vi "test-AsyncMessageWithReplyWithGlobalVariable.vi"(8 "error in (no error)":errorcluster, 11 "TestCase in":refnum<class "testcase-CSMMessage.lvclass">) -> (0 "error out":errorcluster, 3 "TestCase out":refnum<class "testcase-CSMMessage.lvclass">)   [LabVIEW 2017, in "testcase-CSMMessage.lvclass"]
uses:
  testcase-CSMMessage.lvclass
  C:/Program Files (x86)/National Instruments/LabVIEW 2017/vi.lib/addons/_JKI Toolkits/VI Tester/TestCase.llb/TestCase.lvclass
  src/user.lib/_NEVSTOP/Communicable State Machine(CSM)/Communicable State Machine.lvlib
  CSM/Global-TestcaseCSM.vi
  CSM/CSM-Testcase.lvlib
  <vilib>/addons/_JKI Toolkits/VI Tester/TestCase.llb/TestCase.lvclass
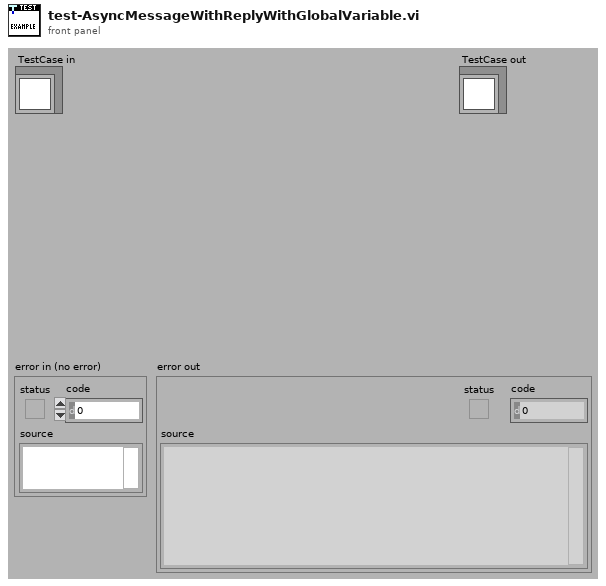
[diagram p1: front panel]
types:
  T1 = cluster{"Arguments":string, "Response":string, "error":errorcluster}
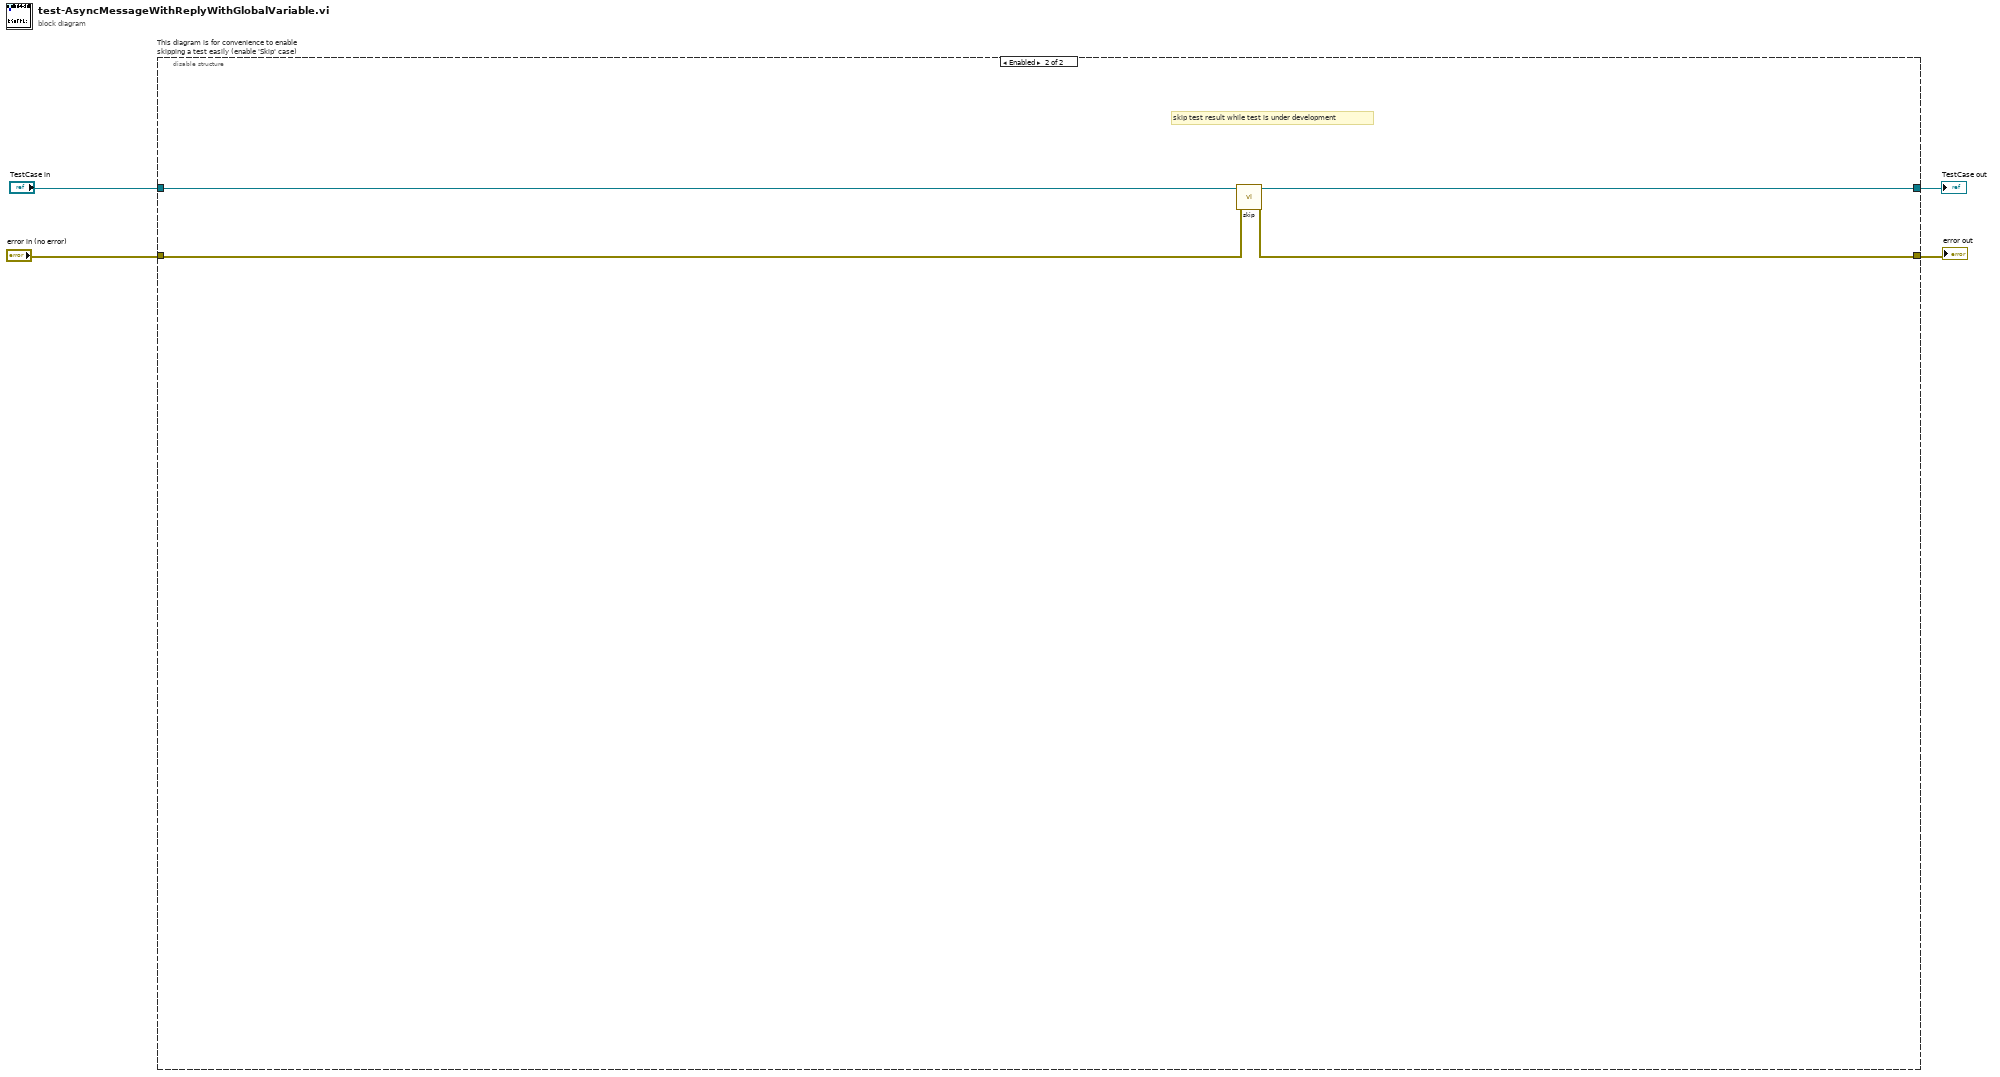
[diagram p0: block diagram]
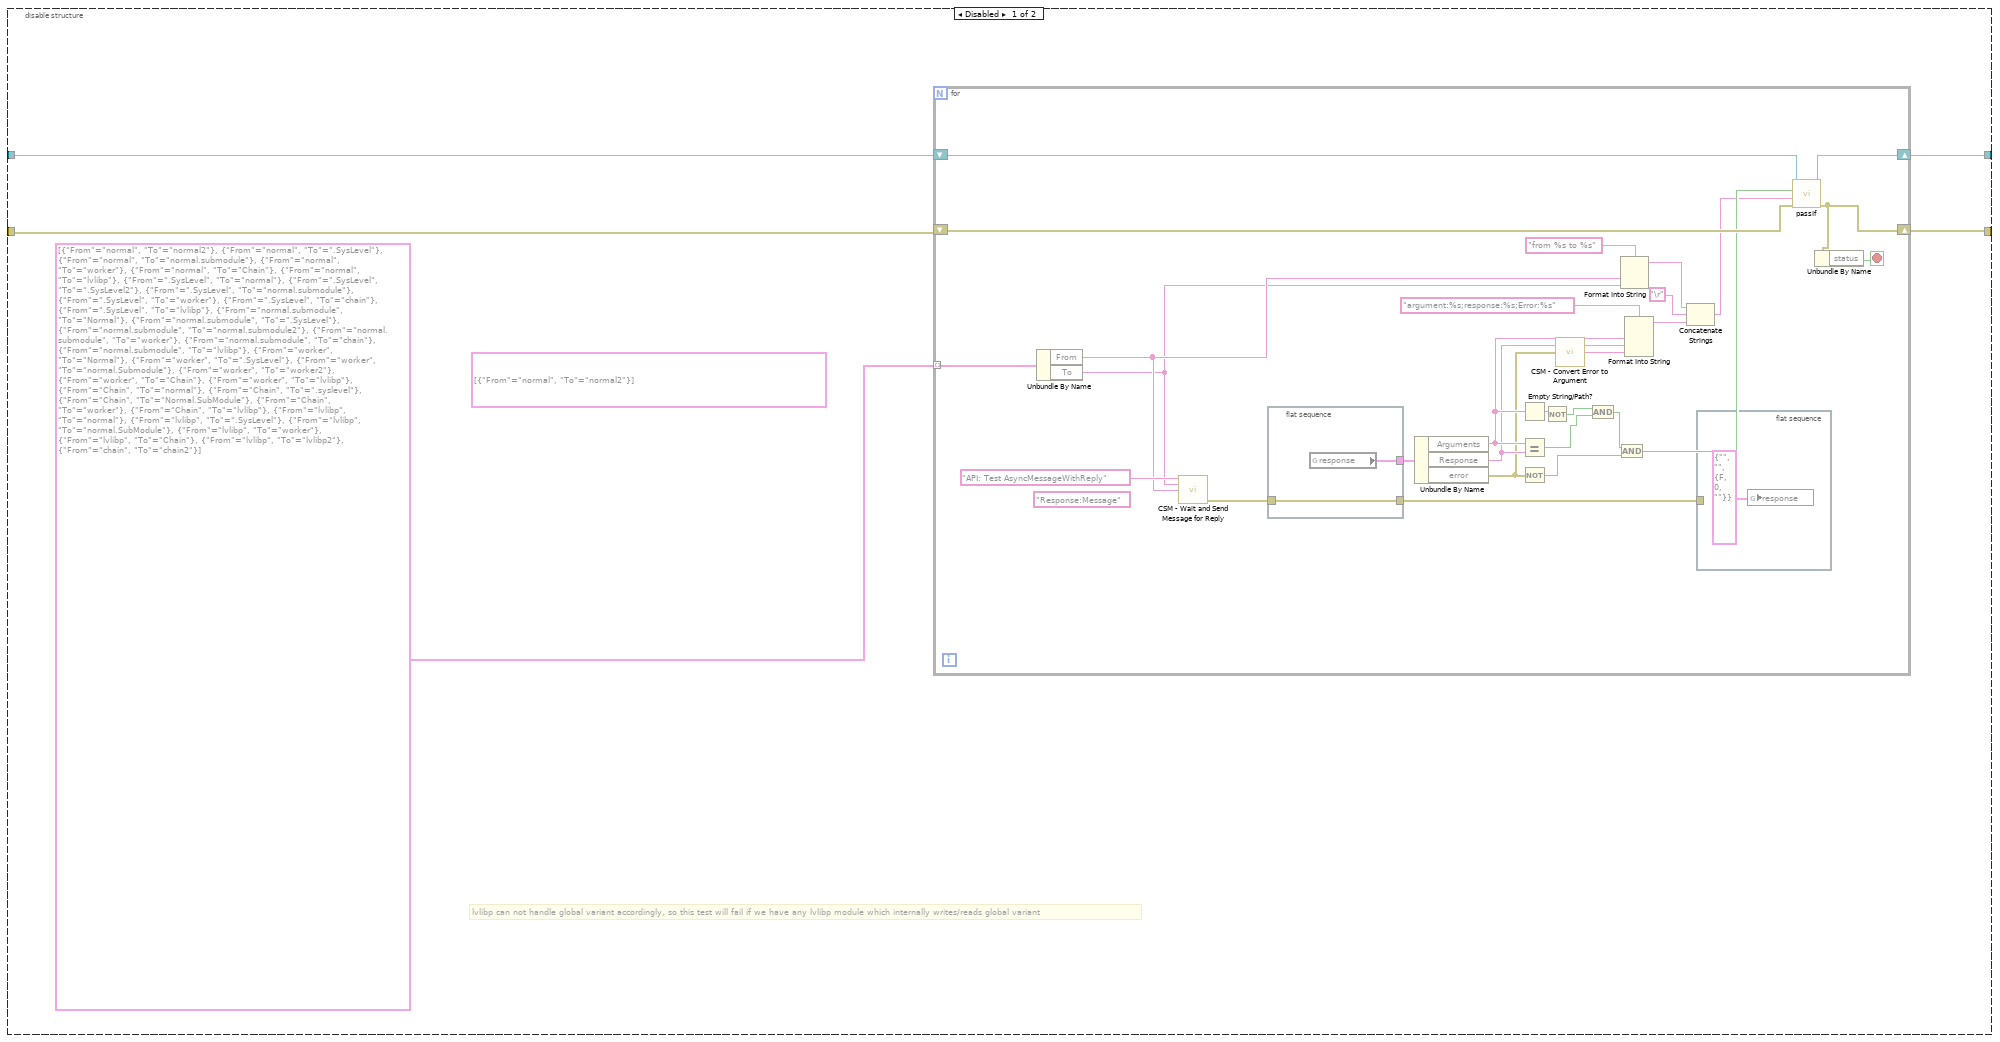
[diagram p2: hidden frame]
diagram:
  n1 = disable-structure "This diagram is for convenience to enable skipping a test easily (enable 'Skip' case)" shown="Enabled" {
    disable-tunnel: "TestCase in" -> [w9 w44]
    disable-tunnel: [w8 w42] -> w1
    disable-tunnel: [w5 w43] -> w3
    disable-tunnel: "error in (no error)" -> [w7 w41]
    frame Disabled {
      (unwired) cluster{"From":string, "To":string}[] [{"From"="normal", "To"="normal2"}]
      # "lvlibp can not handle global variant accordingly, so this test will fail if we have any lvlibp module which internally writes/reads global variant"
      n2 = for {
        tunnel: cluster{"From":string, "To":string}[] [{"From"="normal", "To"="normal2"}, {"From"="normal", "To"=".SysLevel"}, {"From"="normal", "To"="normal.submodule"}, {"From"="normal", "To"="worker"}, {"From"="normal", "To"="Chain"}, {"From"="normal", "To"="lvlibp"}, {"From"=".SysLevel", "To"="normal"}, {"From"=".SysLevel", "To"=".SysLevel2"}, {"From"=".SysLevel", "To"="normal.submodule"}, {"From"=".SysLevel", "To"="worker"}, {"From"=".SysLevel", "To"="chain"}, {"From"=".SysLevel", "To"="lvlibp"}, {"From"="normal.submodule", "To"="Normal"}, {"From"="normal.submodule", "To"=".SysLevel"}, {"From"="normal.submodule", "To"="normal.submodule2"}, {"From"="normal.submodule", "To"="worker"}, {"From"="normal.submodule", "To"="chain"}, {"From"="normal.submodule", "To"="lvlibp"}, {"From"="worker", "To"="Normal"}, {"From"="worker", "To"=".SysLevel"}, {"From"="worker", "To"="normal.Submodule"}, {"From"="worker", "To"="worker2"}, {"From"="worker", "To"="Chain"}, {"From"="worker", "To"="lvlibp"}, {"From"="Chain", "To"="normal"}, {"From"="Chain", "To"=".syslevel"}, {"From"="Chain", "To"="Normal.SubModule"}, {"From"="Chain", "To"="worker"}, {"From"="Chain", "To"="lvlibp"}, {"From"="lvlibp", "To"="normal"}, {"From"="lvlibp", "To"=".SysLevel"}, {"From"="lvlibp", "To"="normal.SubModule"}, {"From"="lvlibp", "To"="worker"}, {"From"="lvlibp", "To"="Chain"}, {"From"="lvlibp", "To"="lvlibp2"}, {"From"="chain", "To"="chain2"}] -> [w32] mode=indexing
        shift-right: [w36] -> w8
        shift-left: w9 -> [w37]
        shift-right: [w13] -> w5
        shift-left: w7 -> [w35]
        stop <- w12 stop-if-true
        (unwired) "Response:Message" ("State")
        n3 = Unbundle By Name(w32) -> ("From"=w11:string, "To"=w10:string)
        n4 = call "CSM - Wait and Send Message for Reply.vi"("State"="API: Test AsyncMessageWithReply", "Arguments (\"\")"=w10, "Target Module"=w11) -> ("error out"=w15:errorcluster)  [unwired: 10 in, 2 out]
        n5 = flat-sequence {
          tunnel: w15 -> [w39]
          tunnel: [w40] -> w17
          tunnel: [w39] -> w16
          frame #0 {
            n6 = global read "Global-TestcaseCSM.vi" "response"() -> (w40:T1)
          }
        }
        n7 = Unbundle By Name(w17) -> ("Arguments"=w26:string, "Response"=w25:string, "error"=w23:errorcluster)
        n8 = Empty String/Path?(string/path=w26) -> (empty?=w30:bool)
        n9 = Equal?(x=w26, y=w25) -> (x = y?=w28:bool)
        n10 = Not(x=w23) -> (.not. x?=w34:bool)
        n11 = Not(x=w30) -> (.not. x?=w29:bool)
        n12 = call "CSM - Convert Error to Argument.vi"("Error"=w23) -> ("Argument"=w24:string)  [unwired: 4 in]
        n13 = And(x=w29, y=w28) -> (x .and. y?=w27:bool)
        n14 = And(x=w27, y=w34) -> (x .and. y?=w33:bool)
        n15 = Format Into String(format string="from %s to %s", w11, w10) -> (resulting string=w19:string)  [unwired: 2 in, 1 out]
        n16 = Format Into String(format string="argument:%s;response:%s;Error:%s", w26, w25, w24) -> (resulting string=w22:string)  [unwired: 2 in, 1 out]
        n17 = Concatenate Strings(w19, "\r", w22) -> (w20:string)
        n18 = flat-sequence {
          tunnel: w16 -> [_]
          frame #0 {
            n19 = global write "Global-TestcaseCSM.vi" "response"(T1 {"Arguments"="", "Response"="", "error"={"status"=FALSE, "code"=0, "source"=""}} ("response")) -> ()
          }
        }
        n20 = call-dynamic "passIf.vi"("error in (no error)"=w35, "message (\"\")"=w20, "pass"=w33, "TestCase in"=w37) -> ("error out"=w13:errorcluster, "TestCase out"=w36:refnum<class "testcase-CSMMessage.lvclass">)  [unwired: 6 in]
        n21 = Unbundle By Name(w13) -> ("status"=w12:bool)
      }
    }
    frame Enabled {
      # "skip test result while test is under development"
      n22 = call <vilib>:"skip.vi"("error in (no error)"=w41, "TestCase in"=w44) -> ("error out"=w43:errorcluster, "TestCase out"=w42:refnum<class "testcase-CSMMessage.lvclass">)  [unwired: 8 in]
    }
  }
  "error out" <- w3
  "TestCase out" <- w1
